vi "File.Check if Exists, If so Inc Name.vi"(8 "error in":errorcluster, 11 "Path":path) -> (0 "error out":errorcluster, 3 "Path Out":path)   [LabVIEW 2024]
uses:
  File Utils.lvlib
panel:
  out "Count":i32
  out "Exists":bool
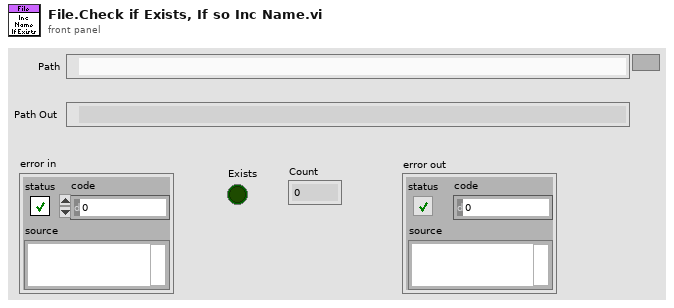
[diagram p1: front panel]
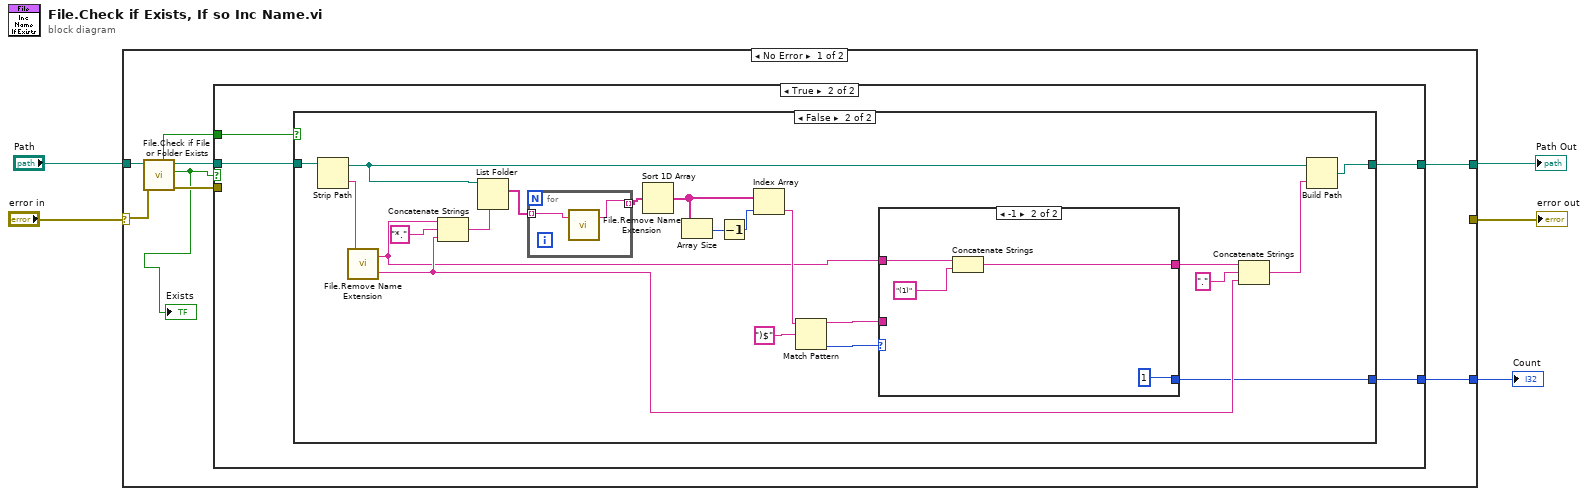
[diagram p0: block diagram]
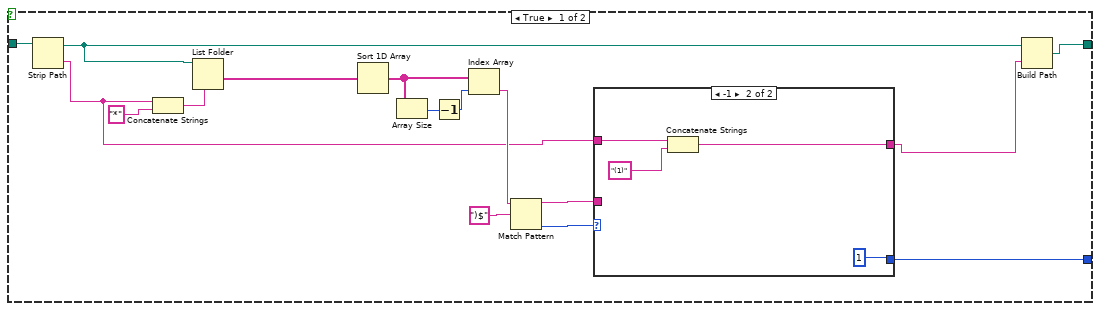
[diagram p3: hidden frame]
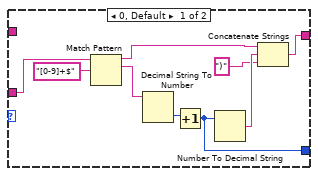
[diagram p4: hidden frame]
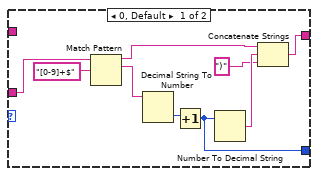
[diagram p5: hidden frame]
diagram:
  n1 = case shown="No Error" "error in" {
    selector: "error in" -> [w10 w85]
    tunnel: "Path" -> [w12 w84]
    tunnel: [_ w85] -> w4
    tunnel: [w9 w84] -> w2
    tunnel: [w7 _] -> w1
    frame No Error {
      n2 = call "File.Check if File or Folder Exists.vi"("error in"=w10, "Path"=w12) -> ("error out"=w11:errorcluster, "Exists"=w8:bool, "Dup Path"=w13:path, "IsDir"=w6:bool)  [unwired: 5 in, 1 out]
      "Exists" <- w8
      n3 = case shown="True" w8 {
        tunnel: w13 -> [w14 w17]
        tunnel: [w14 w18] -> w9
        tunnel: w11 -> [_ _]
        tunnel: [_ w16] -> w7
        tunnel: w6 -> [_ w15]
        frame False {
        }
        frame True {
          n4 = case shown="False" w15 {
            tunnel: [w31 w63] -> w18
            tunnel: w17 -> [w30 w61]
            tunnel: [w22 w49] -> w16
            frame True {
              n5 = Strip Path(path=w30) -> (stripped path=w23:path, name=w20:string)
              n6 = Concatenate Strings(w20, "*" ("string")) -> (w29:string)
              n7 = List Folder(path=w23, pattern=w29) -> (folder names=w21:string[])  [unwired: 2 in, 3 out]
              n8 = Sort 1D Array(array=w21) -> (sorted array=w27:string[])
              n9 = Array Size(array=w27) -> (size(s)=w26:i32)
              n10 = Decrement(x=w26) -> (x-1=w25:i32)
              n11 = Index Array(array=w27, index=w25) -> (element=w24:string)
              n12 = Match Pattern(string=w24, regular expression=")$") -> (before substring=w32:string, offset past match=w33:i32)  [unwired: 1 in, 2 out]
              n13 = case shown="-1" w33 {
                tunnel: [w40 w46] -> w19
                tunnel: w32 -> [w37 _]
                tunnel: [w35 1] -> w22
                tunnel: w20 -> [_ w45]
                frame 0, Default {
                  n14 = Match Pattern(string=w37, regular expression="[0-9]+$") -> (before substring=w38:string, match substring=w42:string)  [unwired: 1 in, 2 out]
                  n15 = Decimal String To Number(string=w42) -> (number=w41:i32)  [unwired: 2 in, 1 out]
                  n16 = Increment(x=w41) -> (x+1=w35:i32)
                  n17 = Number To Decimal String(number=w35) -> (decimal integer string=w39:string)  [unwired: 1 in]
                  n18 = Concatenate Strings(w38, w39, ")") -> (w40:string)
                }
                frame -1 {
                  n19 = Concatenate Strings(w45, "(1)") -> (w46:string)
                }
              }
              n20 = Build Path(base path=w23, name or relative path=w19) -> (appended path=w31:path)
            }
            frame False {
              n21 = Strip Path(path=w61) -> (stripped path=w50:path, name=w60:string)
              n22 = call "File.Remove Name Extension.vi"("File Name"=w60) -> ("Ext"=w57:string, "Name Less Ext"=w48:string)  [unwired: 1 in]
              n23 = Concatenate Strings(w48, "*." ("string"), w57) -> (w59:string)
              n24 = List Folder(path=w50, pattern=w59) -> (filenames=w53:string[])  [unwired: 2 in, 3 out]
              n25 = for {
                tunnel: w53 -> [w70] mode=indexing
                tunnel: [w69] -> w52 mode=indexing
                n26 = call "File.Remove Name Extension.vi"("File Name"=w70) -> ("Name Less Ext"=w69:string)  [unwired: 1 in, 1 out]
              }
              n27 = Sort 1D Array(array=w52) -> (sorted array=w56:string[])
              n28 = Array Size(array=w56) -> (size(s)=w55:i32)
              n29 = Decrement(x=w55) -> (x-1=w54:i32)
              n30 = Index Array(array=w56, index=w54) -> (element=w51:string)
              n31 = Match Pattern(string=w51, regular expression=")$") -> (before substring=w66:string, offset past match=w67:i32)  [unwired: 1 in, 2 out]
              n32 = case shown="-1" w67 {
                tunnel: [w76 w82] -> w65
                tunnel: w66 -> [w73 _]
                tunnel: [w71 1] -> w49
                tunnel: w48 -> [_ w81]
                frame 0, Default {
                  n33 = Match Pattern(string=w73, regular expression="[0-9]+$") -> (before substring=w74:string, match substring=w78:string)  [unwired: 1 in, 2 out]
                  n34 = Decimal String To Number(string=w78) -> (number=w77:i32)  [unwired: 2 in, 1 out]
                  n35 = Increment(x=w77) -> (x+1=w71:i32)
                  n36 = Number To Decimal String(number=w71) -> (decimal integer string=w75:string)  [unwired: 1 in]
                  n37 = Concatenate Strings(w74, w75, ")") -> (w76:string)
                }
                frame -1 {
                  n38 = Concatenate Strings(w81, "(1)") -> (w82:string)
                }
              }
              n39 = Concatenate Strings(w65, ".", w57) -> (w62:string)
              n40 = Build Path(base path=w50, name or relative path=w62) -> (appended path=w63:path)
            }
          }
        }
      }
    }
    frame Error {
    }
  }
  "error out" <- w4
  "Path Out" <- w2
  "Count" <- w1
